vi "audio_play.vi"(6 "Stop":bool, 11 "Bypass":bool) -> ()   [LabVIEW 2018]
uses:
  <vilib>/sound2/lvsound2.llb/Sound Data Format.ctl
  <vilib>/sound2/lvsound2.llb/Sound File Position.ctl
  <vilib>/Analysis/3filter.llb/Filter Passband Type.ctl
  <vilib>/Analysis/4window.llb/windowTd.ctl
  <vilib>/sound2/lvsound2.llb/Sound File Read Open.vi
  <vilib>/sound2/lvsound2.llb/Sound File Read (DBL).vi
  <vilib>/Analysis/3filter.llb/FIR Filter (DBL).vi
  <vilib>/sound2/lvsound2.llb/Sound Output Write (DBL).vi
  <vilib>/Analysis/NI_AALBase.lvlib
  <vilib>/Analysis/NI_AALPro.lvlib
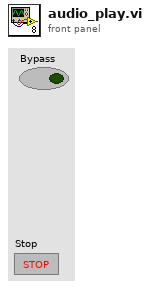
[diagram p1: front panel]
types:
  T1 = typedef "Sound Data Format.ctl" = cluster{"sample rate (S/s)":dbl, "number of channels":i32, "bits per sample":i32}
  T2 = typedef "Sound Output Task ID.ctl" = u32
  T3 = typedef "Sound File Refnum.ctl" = refnum<file>
  T4 = typedef "NI_AALBase.lvlib/Filter Passband Type.ctl" = enum32{"Lowpass", "Highpass", "Bandpass", "Bandstop"}
  T5 = typedef "NI_AALPro.lvlib/windowTd.ctl" = u32
  T6 = typedef "Sound File Position.ctl" = u16
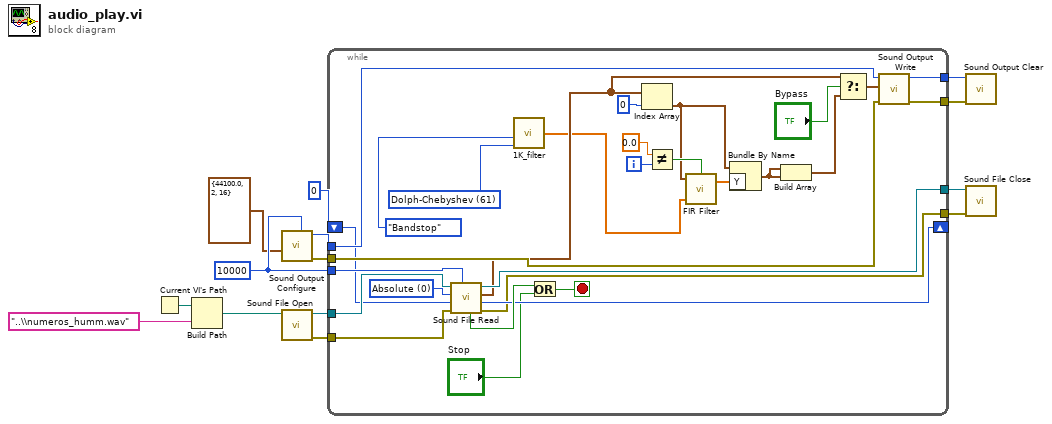
[diagram p0: block diagram]
diagram:
  w11 = 10000 ("number of samples/ch")
  n1 = Current VI's Path() -> (path=w1:path)
  n2 = Build Path(base path=w1, name or relative path="..\\numeros_humm.wav") -> (appended path=w2:path)
  n3 = call <vilib>:"Sound Output Configure.vi"("number of samples/ch"=w11, "sound format"=T1 {"sample rate (S/s)"=44100.0, "number of channels"=2, "bits per sample"=16}) -> ("error out"=w5:errorcluster, "task ID"=w7:T2)  [unwired: 8 in]
  n4 = call-poly <vilib>:"Sound File Open.vi"("path"=w2) -> ("error out"=w12:errorcluster, "sound file refnum"=w9:T3)  [unwired: 9 in]
  n5 = while {
    tunnel: w5 -> [w43]
    tunnel: [w42] -> w6
    tunnel: w7 -> [w41]
    tunnel: [w40] -> w8
    tunnel: w9 -> [w39]
    tunnel: [w38] -> w10
    tunnel: w11 -> [w35]
    shift-right: [w33] -> _
    shift-left: 0 ("offset") -> [w32]
    tunnel: w12 -> [w31]
    tunnel: [w30] -> w13
    i -> [w26]
    stop <- w37 stop-if-true
    w15 = T5 61 items=["Rectangle"=0, "Hanning"=1, "Hamming"=2, "Blackman-Harris"=3, "Exact Blackman"=4, "Blackman"=5, "Flat Top"=6, "4 Term B-Harris "=7, "7 Term B-Harris"=8, "Low Sidelobe"=9, "Blackman Nuttall"=11, "Triangle"=30, "Bartlett-Hanning"=31, "Bohman"=32, "Parzen"=33, "Welch"=34, "Kaiser"=60, "Dolph-Chebyshev"=61, "Gaussian"=62] ("Ventana")
    w34 = T6 0 items=["Absolute"=0, "Relative"=2] ("position mode")
    n6 = call-poly <vilib>:"Sound File Read.vi"("number of samples/ch (-1: all)"=w35, "error in (no error)"=w31, "position offset"=w32, "position mode"=w34, "sound file refnum"=w39) -> ("error out"=w30:errorcluster, "offset"=w33:i32, "data"=w24:waveform(dbl)[], "sound file refnum out"=w38:T3, "end of file?"=w36:bool)  [unwired: 2 in]
    n7 = call "1K_filter.vi"("filter type"=Filter_Passband_Type."Bandstop", "Ventana"=w15) -> ("FIR Windowed Coefficients"=w17:dbl[])  [unwired: 3 in]
    n8 = Or(x=w36, y="Stop") -> (x .or. y?=w37:bool)
    n9 = Index Array(array=w24, index=0) -> (element=w20:waveform(dbl))
    n10 = Not Equal?(x=0.0, y=w26) -> (x != y?=w25:bool)
    n11 = call-poly <vilib>:"FIR Filter.vi"("init/cont (init:F)"=w25, "FIR Coefficients"=w17, "X"=w20) -> ("Filtered X"=w29:dbl[])  [unwired: 1 in, 1 out]
    n12 = Bundle By Name(cluster=w20, "Y"=w29) -> (w18:waveform(dbl))
    n13 = Build Array(w18, w18) -> (w22:waveform(dbl)[])
    n14 = Select(t=w24, s="Bypass", f=w22) -> (s? t:f=w23:waveform(dbl)[])
    n15 = call-poly <vilib>:"Sound Output Write.vi"("error in (no error)"=w43, "data"=w23, "task ID"=w41) -> ("error out"=w42:errorcluster, "task ID out"=w40:T2)  [unwired: 7 in]
  }
  n16 = call <vilib>:"Sound Output Clear.vi"("error in (no error)"=w6, "task ID"=w8) -> ()  [unwired: 9 in, 1 out]
  n17 = call <vilib>:"Sound File Close.vi"("error in (no error)"=w13, "sound file refnum"=w10) -> ()  [unwired: 9 in, 1 out]
